vi "GW_Block_Move.vi"(7 "站點(記錄用)":string="790", 8 "error in (no error)":errorcluster, 10 "Workplace_id":i16, 11 "DBLink":string) -> (0 "error out":errorcluster, 2 "[glue_data_id]":string)   [LabVIEW 2019]
panel:
  # "此id為該位置檔快放行，把資料移至移動中"
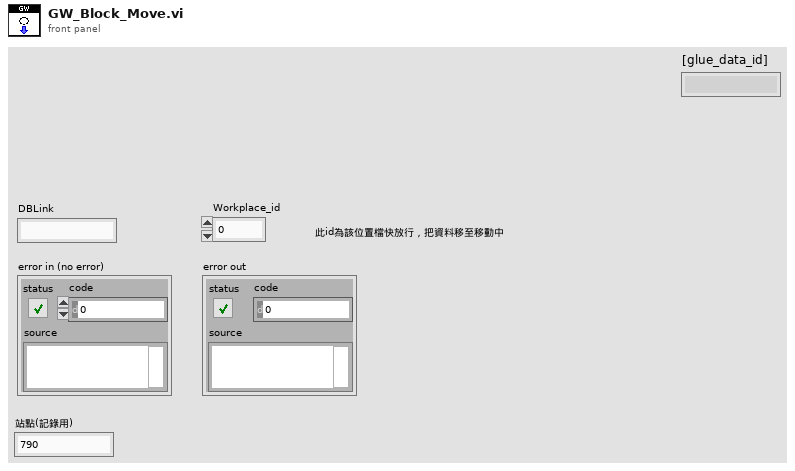
[diagram p1: front panel]
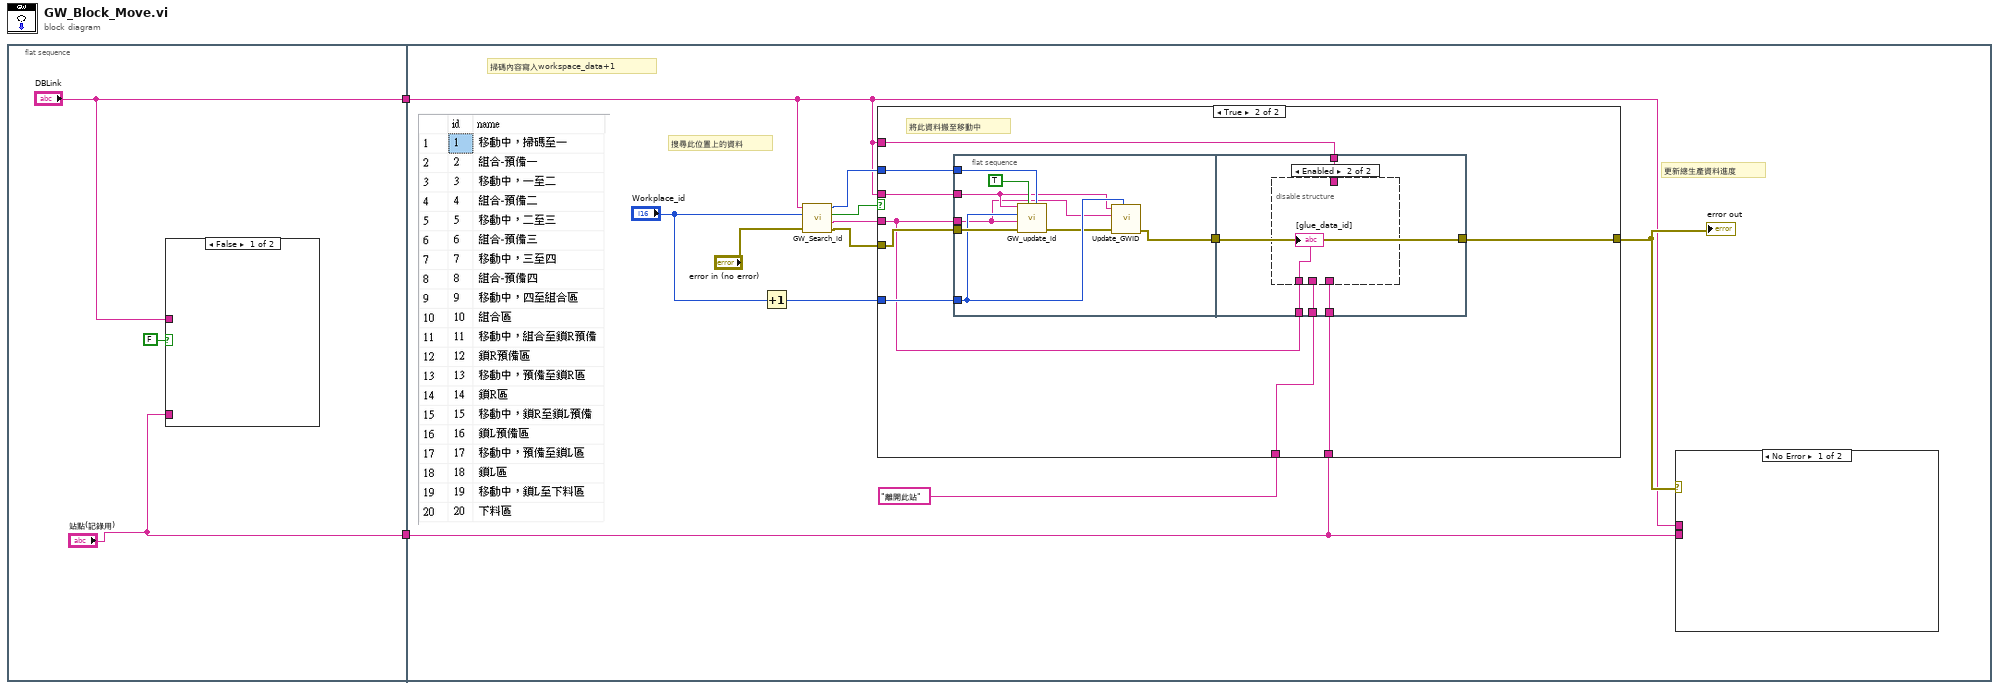
[diagram p0: block diagram]
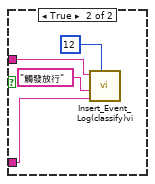
[diagram p2: hidden frame]
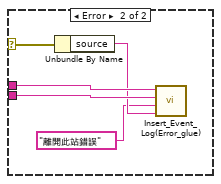
[diagram p3: hidden frame]
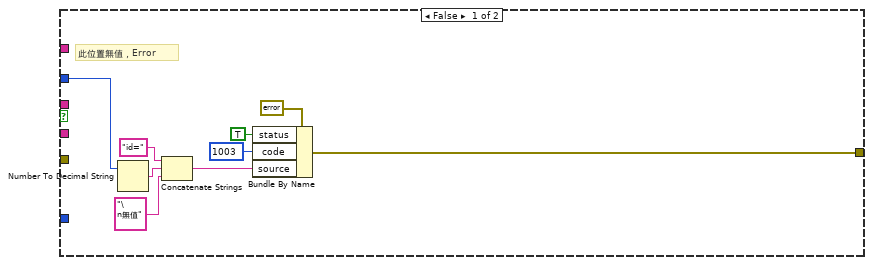
[diagram p4: hidden frame]
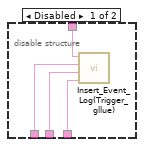
[diagram p5: hidden frame]
diagram:
  n1 = flat-sequence {
    tunnel: ["DBLink"] -> w2
    tunnel: ["站點(記錄用)"] -> w1
    tunnel: w2 -> [w11]
    tunnel: w1 -> [w10]
    frame #0 {
      n2 = case shown="False" FALSE {
        tunnel: "DBLink" -> [_ w7]
        tunnel: "站點(記錄用)" -> [_ w6]
        frame False {
        }
        frame True {
          n3 = call "Insert_Event_Log(classify)vi.vi"("classify"=i16 12, "data"=w6, "message"="觸發放行", "DBlink"=w7) -> ()  [unwired: 7 in, 1 out]
        }
      }
    }
    frame #1 {
      # "搜尋此位置上的資料"
      # "更新總生產資料進度"
      # "掃碼內容寫入workspace_data+1"
      n4 = Increment(x="Workplace_id") -> (x+1=w20:i16)
      n5 = call "GW_Search_id.vi"("error in (no error)"="error in (no error)", "id"="Workplace_id", "DBlink"=w11) -> ("error out"=w14:errorcluster, "[glue_data_id]"=w15:string, "找到"=w16:bool, "取得ID"=w17:i16)  [unwired: 5 in]
      n6 = case shown="True" w16 {
        tunnel: w11 -> [_ w40]
        tunnel: w15 -> [_ w37]
        tunnel: w14 -> [_ w44]
        tunnel: w17 -> [w31 w43]
        tunnel: w20 -> [_ w41]
        tunnel: [w26 w42] -> w13
        tunnel: "離開此站" ("message") -> [_ w35]
        tunnel: w10 -> [_ w36]
        tunnel: w11 -> [_ w38]
        frame False {
          # "此位置無值，Error"
          n7 = Number To Decimal String(number=w31) -> (decimal integer string=w29:string)  [unwired: 1 in]
          n8 = Concatenate Strings("id=", w29, "\n無值" ("string")) -> (w27:string)
          n9 = Bundle By Name(cluster=errorcluster {"status"=FALSE, "code"=0, "source"=""} ("error out"), "status"=TRUE, "code"=1003, "source"=w27) -> (w26:errorcluster)
        }
        frame True {
          # "將此資料搬至移動中"
          n10 = flat-sequence {
            tunnel: w44 -> [w52]
            tunnel: w43 -> [w50]
            tunnel: w41 -> [w48]
            tunnel: w40 -> [w46]
            tunnel: w37 -> [w45]
            tunnel: [w49] -> w39
            tunnel: [w57] -> w42
            tunnel: w39 -> [w57]
            tunnel: w38 -> [w56]
            tunnel: w37 -> [w55]
            tunnel: w36 -> [w53]
            tunnel: w35 -> [w54]
            frame #0 {
              n11 = call "GW_update_id.vi"("NULL: workplace_id"=w50, "Set null"=TRUE, "error in (no error)"=w52, "glue_data_id"=w45, "id"=w48, "DBlink"=w46) -> ("error out"=w47:errorcluster)  [unwired: 5 in]
              n12 = call "Update_GWID .vi"("[glue_workspace_id]"=w48, "error in (no error)"=w47, "[glue_data_id]"=w45, "DBlink"=w46) -> ("error out"=w49:errorcluster)  [unwired: 7 in]
            }
            frame #1 {
              n13 = disable-structure shown="Enabled" {
                disable-tunnel: w56 -> [w61 _]
                disable-tunnel: w55 -> [w60 w62]
                disable-tunnel: w54 -> [w59 _]
                disable-tunnel: w53 -> [w58 _]
                frame Disabled {
                  n14 = call "Insert_Event_Log(Trigger_gllue).vi"("data"=w58, "message"=w59, "id"=w60, "DBlink"=w61) -> ()  [unwired: 8 in]
                }
                frame Enabled {
                  "[glue_data_id]" <- w62
                }
              }
            }
          }
        }
      }
      "error out" <- w13
      n15 = case shown="No Error" w13 {
        selector: w13 -> [_ w23]
        tunnel: w11 -> [_ w25]
        tunnel: w10 -> [_ w24]
        frame No Error {
        }
        frame Error {
          n16 = Unbundle By Name(w23) -> ("source"=w22:string)
          n17 = call "Insert_Event_Log(Error_glue).vi"("data"=w22, "message"="離開此站錯誤", "id"=w24, "DBlink"=w25) -> ()  [unwired: 8 in]
        }
      }
    }
  }
